vi "Actor Core.vi"(8 "error in":errorcluster, 11 "Sim Sensor Interface Actor in":refnum<class "Sim Sensor Interface Actor.lvclass">) -> (0 "error out":errorcluster, 3 "Actor out":refnum<class "Actor.lvclass">)   [LabVIEW 2022 SP3, in "Sim Sensor Interface Actor.lvlib" / "Sim Sensor Interface Actor.lvclass"]
doc: "(<B>Filename</B>: Actor Framework.lvlib:Actor.lvclass:Actor Core.vi)\n\nReceives messages to the actor, reacts to them, and initiates any error handling that may shut the actor down.\n\nDescendant classes may override this VI to append parallel tasks for the actor to complete while it handles messages. Overrides use the Call Parent Class Method node."
uses:
  Sim Sensor Interface Actor.lvclass
  Sim Sensor Interface Actor.lvclass/Sim Sensor Interface Actor.ctl
  <vilib>/ActorFramework/Stop Msg/Stop Msg.lvclass
  <vilib>/ActorFramework/Actor/Actor.lvclass
  Sim User Console Actor/Abstract User Console Actor/Sim User Console Actor.lvclass
  Abstract Sensor Interface Actor/Abstract Sensor Interface Actor/Abstract Sensor Interface Actor.lvclass
  C:/Workspace/CLA/Elevator AF_2022/Abstract Sensor Interface Actor/Abstract Sensor Interface Actor/Abstract Sensor Interface Actor.lvclass
  C:/Program Files/National Instruments/LabVIEW 2022/vi.lib/ActorFramework/Actor/Actor.lvclass
  C:/Workspace/CLA/Elevator AF_2022/Sim Sensor Interface Actor/Sim Sensor Interface Actor/Sim Sensor Interface Actor.lvclass
panel:
  in  "Elevator Position":u32(slide) scale=1.0..4.0
  # "[Covers: UI4] \n[Covers: UI4A]"
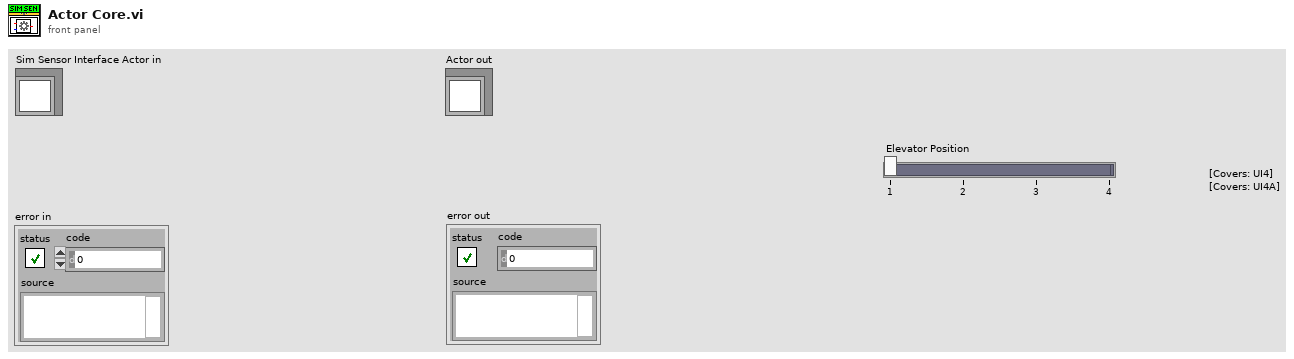
[diagram p1: front panel]
types:
  T1 = enum8{"Enabled", "Disabled", "Disabled and Grayed Out"}
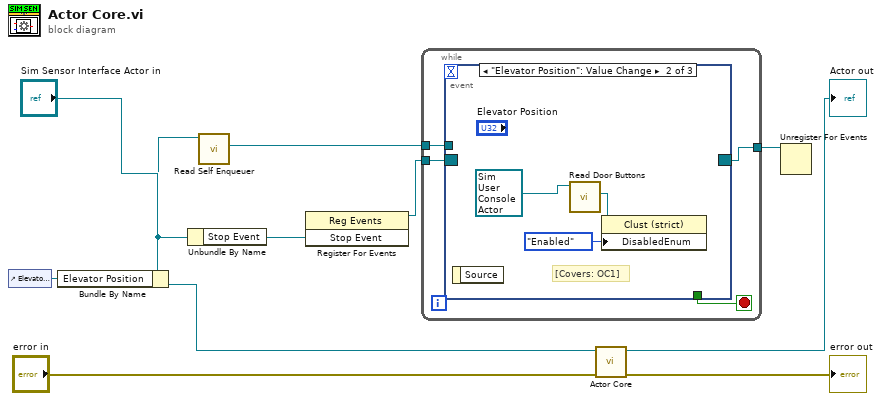
[diagram p0: block diagram]
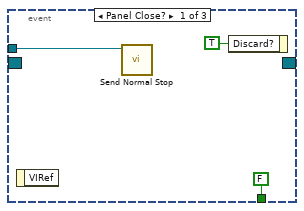
[diagram p2: hidden frame]
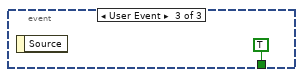
[diagram p3: hidden frame]
diagram:
  n1 = control-ref of="Elevator Position"() -> (w5:refnum<vi>)
  n2 = Bundle By Name(cluster="Sim Sensor Interface Actor in", "Elevator Position"=w5) -> (w3:refnum<class "Sim Sensor Interface Actor.lvclass">)
  n3 = Unbundle By Name(w3) -> ("Stop Event"=w4:refnum<user-event>)
  n4 = call <vilib>:"Read Self Enqueuer.vi"("Actor"=w3) -> ("Self Enqueuer"=w6:refnum<class "Message Enqueuer.lvclass">)  [unwired: 10 in]
  n5 = register-events(w4) -> (reference out=w2:refnum<event-registration>)  [unwired: 2 in, 1 out]
  n6 = while {
    tunnel: w6 -> [w13]
    tunnel: w2 -> [w12]
    tunnel: [w11] -> w1
    stop <- w14 stop-if-true
    n7 = event shown="[1] \"Elevator Position\": Value Change" {
      selector: w12 -> [_ _ _]
      dyn-events: [_ _ _] -> w11
      timeout: _ -> [_ _ _]
      tunnel: [FALSE _ TRUE] -> w14
      tunnel: w13 -> [w15 _ _]
      event Panel Close? {
        n8 = event-data() -> ()  [unwired: 1 in, 1 out]
        n9 = call <vilib>:"Send Normal Stop.vi"("Message Enqueuer"=w15) -> ()  [unwired: 10 in, 1 out]
        n10 = event-data("Discard?"=TRUE) -> ()  [unwired: 1 in, 1 out]
      }
      event "Elevator Position": Value Change {
        # "[Covers: OC1]"
        n11 = event-data() -> ()  [unwired: 1 in, 1 out]
        n12 = call "Read Door Buttons.vi"("Sim User Console Actor in"=refnum<class "Sim User Console Actor.lvclass"> refnum ("Sim User Console Actor.lvlib:Sim User Console Actor.lvclass")) -> ("Door Buttons"=w20:refnum<vi>)  [unwired: 8 in, 2 out]
        n13 = property class="Clust (strict)"(reference=w20, "DisabledEnum"=T1."Enabled" ("Disabled")) -> ()  [unwired: 1 in, 2 out]
      }
      event User Event {
        n14 = event-data() -> ()  [unwired: 1 in, 1 out]
      }
    }
  }
  n15 = call-parent "Actor Core.vi"("error in"="error in", "Actor in"=w3) -> ("error out"=→"error out":errorcluster, "Actor out"=→"Actor out":refnum<class "Actor.lvclass">)  [unwired: 8 in]
  n16 = Unregister For Events(event registration refnum=w1) -> ()  [unwired: 1 in, 1 out]
